vi "_041.vi"() -> ()   [LabVIEW 2024]
uses:
  System.Speech
panel:
  in  "textToSpeak":string
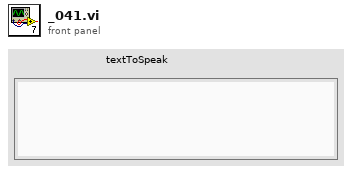
[diagram p1: front panel]
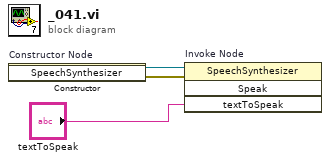
[diagram p0: block diagram]
diagram:
  n1 = constructor on="Constructor Node" class="SpeechSynthesizer"() -> (reference out=w3:refnum<k24>, error out=w2:errorcluster)  [unwired: 3 in, 1 out]
  n2 = invoke on="Invoke Node" class="SpeechSynthesizer" method="Speak"(reference=w3, error in=w2, "textToSpeak"="textToSpeak") -> ()  [unwired: 1 in, 4 out]
